vi "cubic.vi"(8 "path":bool, 9 "h":dbl, 10 "y":dbl, 11 "x":dbl) -> (0 "path_y 2":dbl[](array[numeric]), 1 "path_x 2":dbl[](array[numeric]), 2 "b":dbl, 3 "a":dbl)   [LabVIEW 2012]
uses:
  <vilib>/Analysis/Matrix/Numeric/Conversions/Array To Matrix - RA2.vi
  <vilib>/Analysis/Matrix/Numeric/Conversions/Array To Matrix - RA.vi
  <vilib>/Analysis/Matrix/Numeric/Multiply/Multiply - RM,RM.vi
  <vilib>/Analysis/Matrix/NI_Matrix.lvlib
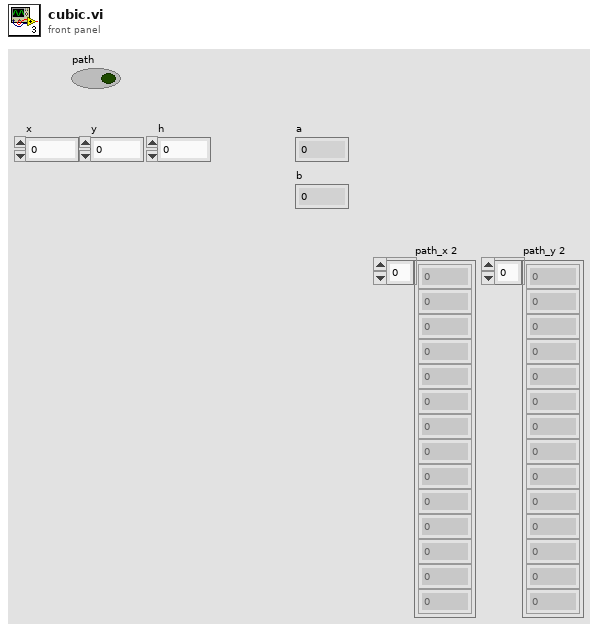
[diagram p1: front panel]
types:
  T1 = typedef "NI_Matrix.lvlib/RealMatrix.ctl" = dbl[][]
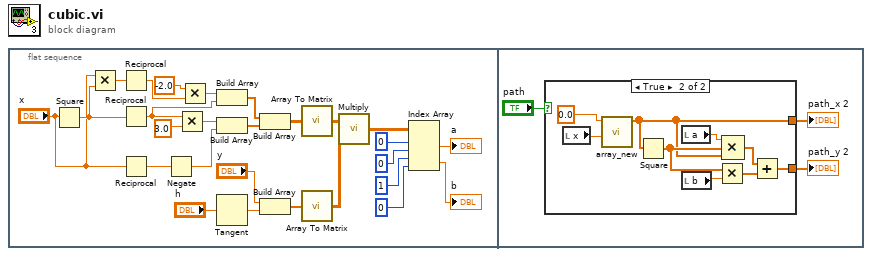
[diagram p0: block diagram]
diagram:
  n1 = flat-sequence {
    frame #0 {
      n2 = Square(x="x") -> (x^2=w8:dbl)
      n3 = Multiply(x="x", y=w8) -> (x*y=w7:dbl)
      n4 = Reciprocal(x=w7) -> (1/x=w9:dbl)
      n5 = Reciprocal(x=w8) -> (1/x=w12:dbl)
      n6 = Reciprocal(x="x") -> (1/x=w15:dbl)
      n7 = Negate(x=w15) -> (-x=w16:dbl)
      n8 = Multiply(x=w12, y=3.0) -> (x*y=w14:dbl)
      n9 = Multiply(x=-2.0, y=w9) -> (x*y=w11:dbl)
      n10 = Build Array(w11, w12) -> (w17:dbl[])
      n11 = Build Array(w14, w16) -> (w18:dbl[])
      n12 = Tangent(1:"h") -> (0:w3:dbl)
      n13 = Build Array(w17, w18) -> (w19:dbl[][])
      n14 = Build Array("y", w3) -> (w21:dbl[])
      n15 = call-poly <vilib>:"Array To Matrix.vi"("Real 2D Array"=w19) -> ("Real Matrix"=w20:T1)
      n16 = call-poly <vilib>:"Array To Matrix.vi"("Real 1D Array"=w21) -> ("Real Matrix (Column Vector)"=w22:T1)
      n17 = call-poly <vilib>:"Multiply.vi"("Real Matrix B"=w22, "Real Matrix A"=w20) -> ("A * B"=w23:T1)
      n18 = Index Array(array=w23, index (row) #1=0 ("index (row)"), index (col) #1=0 ("disabled index (col)"), index (row) #2=1 ("index (row)"), index (col) #2=0 ("disabled index (col)")) -> (element #1=→"a":dbl, element #2=→"b":dbl)
    }
    frame #1 {
      n19 = case shown="True" "path" {
        tunnel: [_ w32] -> w29
        tunnel: [_ w31] -> w28
        frame False {
        }
        frame True {
          n20 = local read "x"() -> (w35:dbl)
          n21 = call "array_new.vi"("end"=w35, "start"=0.0) -> ("Array"=w31:dbl[])  [unwired: 8 in, 1 out]
          n22 = Square(x=w31) -> (x^2=w37:dbl[])
          n23 = local read "a"() -> (w34:dbl)
          n24 = local read "b"() -> (w33:dbl)
          n25 = Multiply(x=w37, y=w33) -> (x*y=w39:dbl[])
          n26 = Compound Arithmetic op=MULTIPLY(w34, w37, w31) -> (w38:dbl[])
          n27 = Add(x=w38, y=w39) -> (x+y=w32:dbl[])
        }
      }
      "path_x 2" <- w28
      "path_y 2" <- w29
    }
  }
